vi "20220107_HW00.vi"() -> ()   [LabVIEW 2019]
uses:
  WaveData.ctl
panel:
  out "Graph":dbl[][](graph)
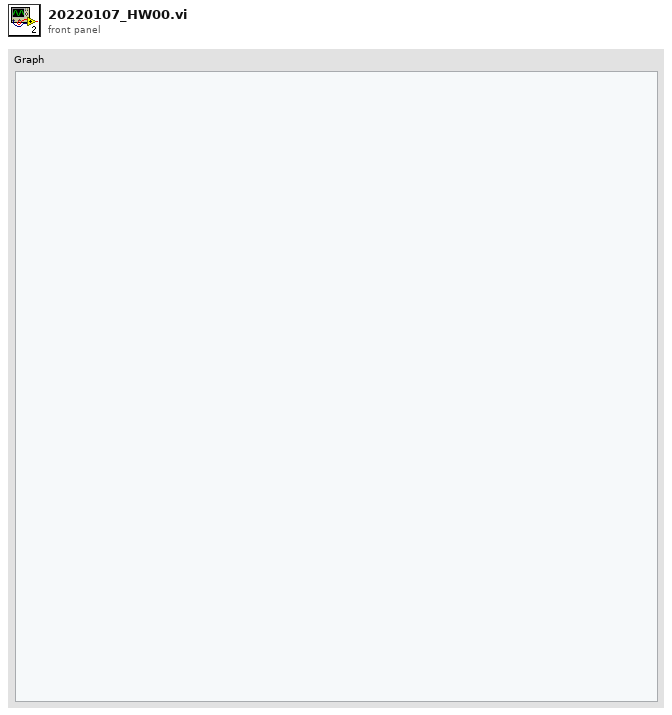
[diagram p1: front panel]
types:
  T1 = typedef "WaveData.ctl" = cluster{"Begin Time":u32, "XY":cluster{"X":dbl, "Y":dbl}}
  T2 = typedef "LVPoint32TypeDef.ctl" = cluster{"Horizontal":i32, "Vertical":i32}
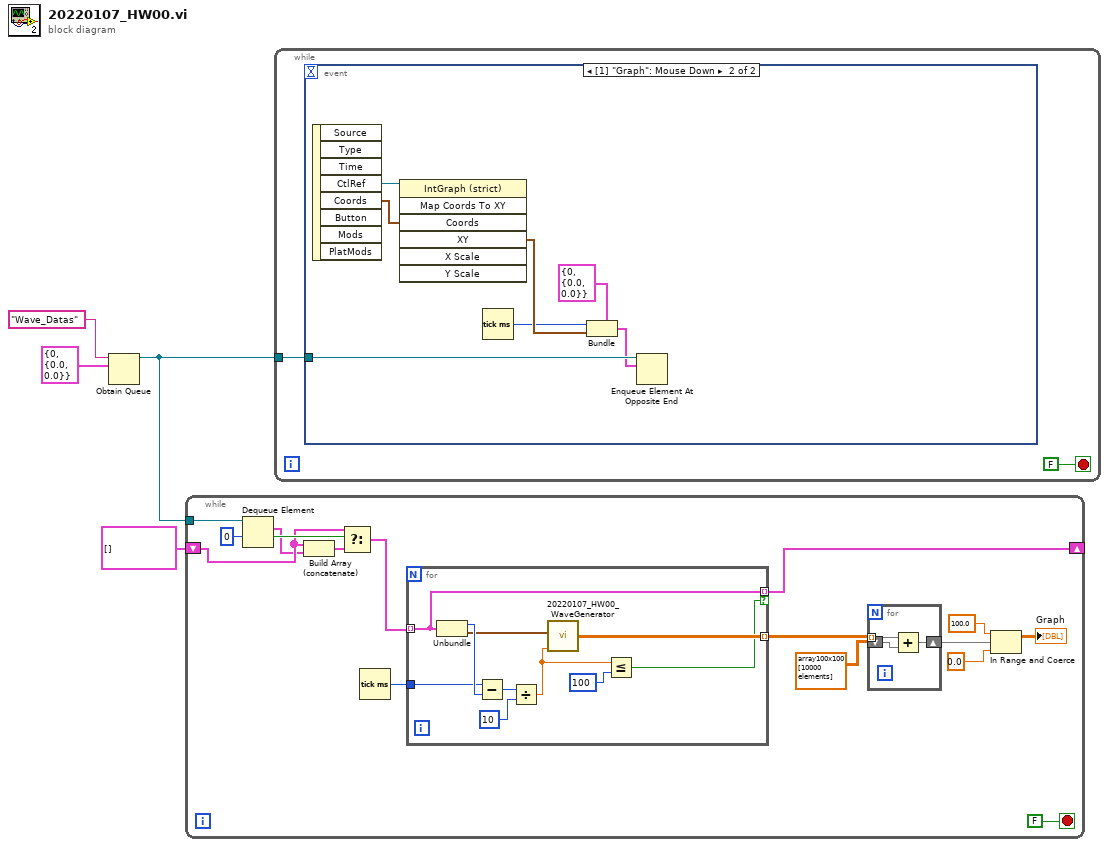
[diagram p0: block diagram]
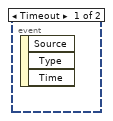
[diagram p2: hidden frame]
diagram:
  n1 = Obtain Queue(name (unnamed)="Wave_Datas", element data type=T1 {"Begin Time"=0, "XY"={"X"=0.0, "Y"=0.0}} ("Wave Data")) -> (queue out=w3:refnum<queue>)  [unwired: 3 in, 2 out]
  n2 = while {
    tunnel: w3 -> [w17]
    shift-right: [w9] -> _
    shift-left: T1[] [] -> [w13]
    stop <- FALSE stop-if-true
    n3 = Dequeue Element(queue=w17, timeout in ms (-1)=0) -> (element=w12:T1, timed out?=w14:bool)  [unwired: 1 in, 2 out]
    n4 = Build Array (concatenate)(w13, w12) -> (w15:T1[])
    n5 = Select(t=w13, s=w14, f=w15) -> (s? t:f=w11:T1[])
    n6 = Tick Count (ms)() -> (millisecond timer value=w10:u32)
    n7 = for {
      tunnel: [w33] -> w19 mode=indexing
      tunnel: w11 -> [w25] mode=indexing
      tunnel: w10 -> [w28]
      tunnel: [w25] -> w9 mode=indexing if=w24
      n8 = Unbundle(w25) -> ("Begin Time"=w30:u32, "XY"=w29:cluster{"X":dbl, "Y":dbl})
      n9 = Subtract(x=w28, y=w30) -> (x-y=w32:u32)
      n10 = Divide(x=w32, y=u32 10) -> (x/y=w27:dbl)
      n11 = call "20220107_HW00_WaveGenerator.vi"("Time"=w27, "Coords"=w29) -> ("Graph"=w33:dbl[][])  [unwired: 2 in]
      n12 = Less Or Equal?(x=w27, y=u32 100) -> (x <= y?=w24:bool)
    }
    n13 = for {
      tunnel: w19 -> [w23] mode=indexing
      shift-right: [w22] -> w8
      shift-left: dbl[][] array100x100[10000 elements] -> [w21]
      n14 = Add(x=w23, y=w21) -> (x+y=w22:dbl[][])
    }
    n15 = In Range and Coerce(upper limit=100.0, x=w8, lower limit=0.0) -> (coerced(x)=→"Graph":dbl[][])  [unwired: 1 out]
  }
  n16 = while {
    tunnel: w3 -> [w34]
    stop <- FALSE stop-if-true
    n17 = event shown="[1] \"Graph\": Mouse Down" {
      selector: _ -> [_ _]
      dyn-events: _ -> [_ _]
      timeout: _ -> [_ _]
      tunnel: w34 -> [_ w38]
      event Timeout {
        n18 = event-data() -> ()  [unwired: 1 in, 3 out]
      }
      event "Graph": Mouse Down {
        n19 = event-data() -> ("CtlRef"=w42:refnum<vi>, "Coords"=w41:T2)  [unwired: 1 in, 6 out]
        n20 = invoke class="IntGraph (strict)" method="Map Coords To XY"(reference=w42, "Coords"=w41) -> ("XY"=w39:cluster{"X":dbl, "Y":dbl})  [unwired: 5 in, 6 out]
        n21 = Tick Count (ms)() -> (millisecond timer value=w36:u32)
        n22 = Bundle(cluster=T1 {"Begin Time"=0, "XY"={"X"=0.0, "Y"=0.0}} ("Wave Data"), "Begin Time"=w36, "XY"=w39) -> (w37:T1)
        n23 = Enqueue Element At Opposite End(queue=w38, element=w37) -> ()  [unwired: 2 in, 3 out]
      }
    }
  }
